vi "HW2.vi"() -> ()   [LabVIEW 2021]
panel:
  out "Key Pressed":i16
  out "turn":dbl
  out "Vref":dbl
  in  "Send value 7":dbl
  in  "Vref":dbl
  in  "Send value 8":dbl
  in  "Send value 6":dbl
  in  "Send value 5":dbl
  in  "Send value 4":dbl
  in  "Send value 3":dbl
  in  "turn":dbl
  in  "Send button":bool
  out "RecvValue 8":dbl
  out "RecvValue 7":dbl
  out "RecvValue 6":dbl
  out "RecvValue 5":dbl
  out "RecvValue 4":dbl
  out "RecvValue 3":dbl
  out "Y":dbl
  out "X":dbl
  in  "Display History":bool
  in  "Size of Rectangle":i16=20
  in  "Stop":bool
  out "2D Picture":picture
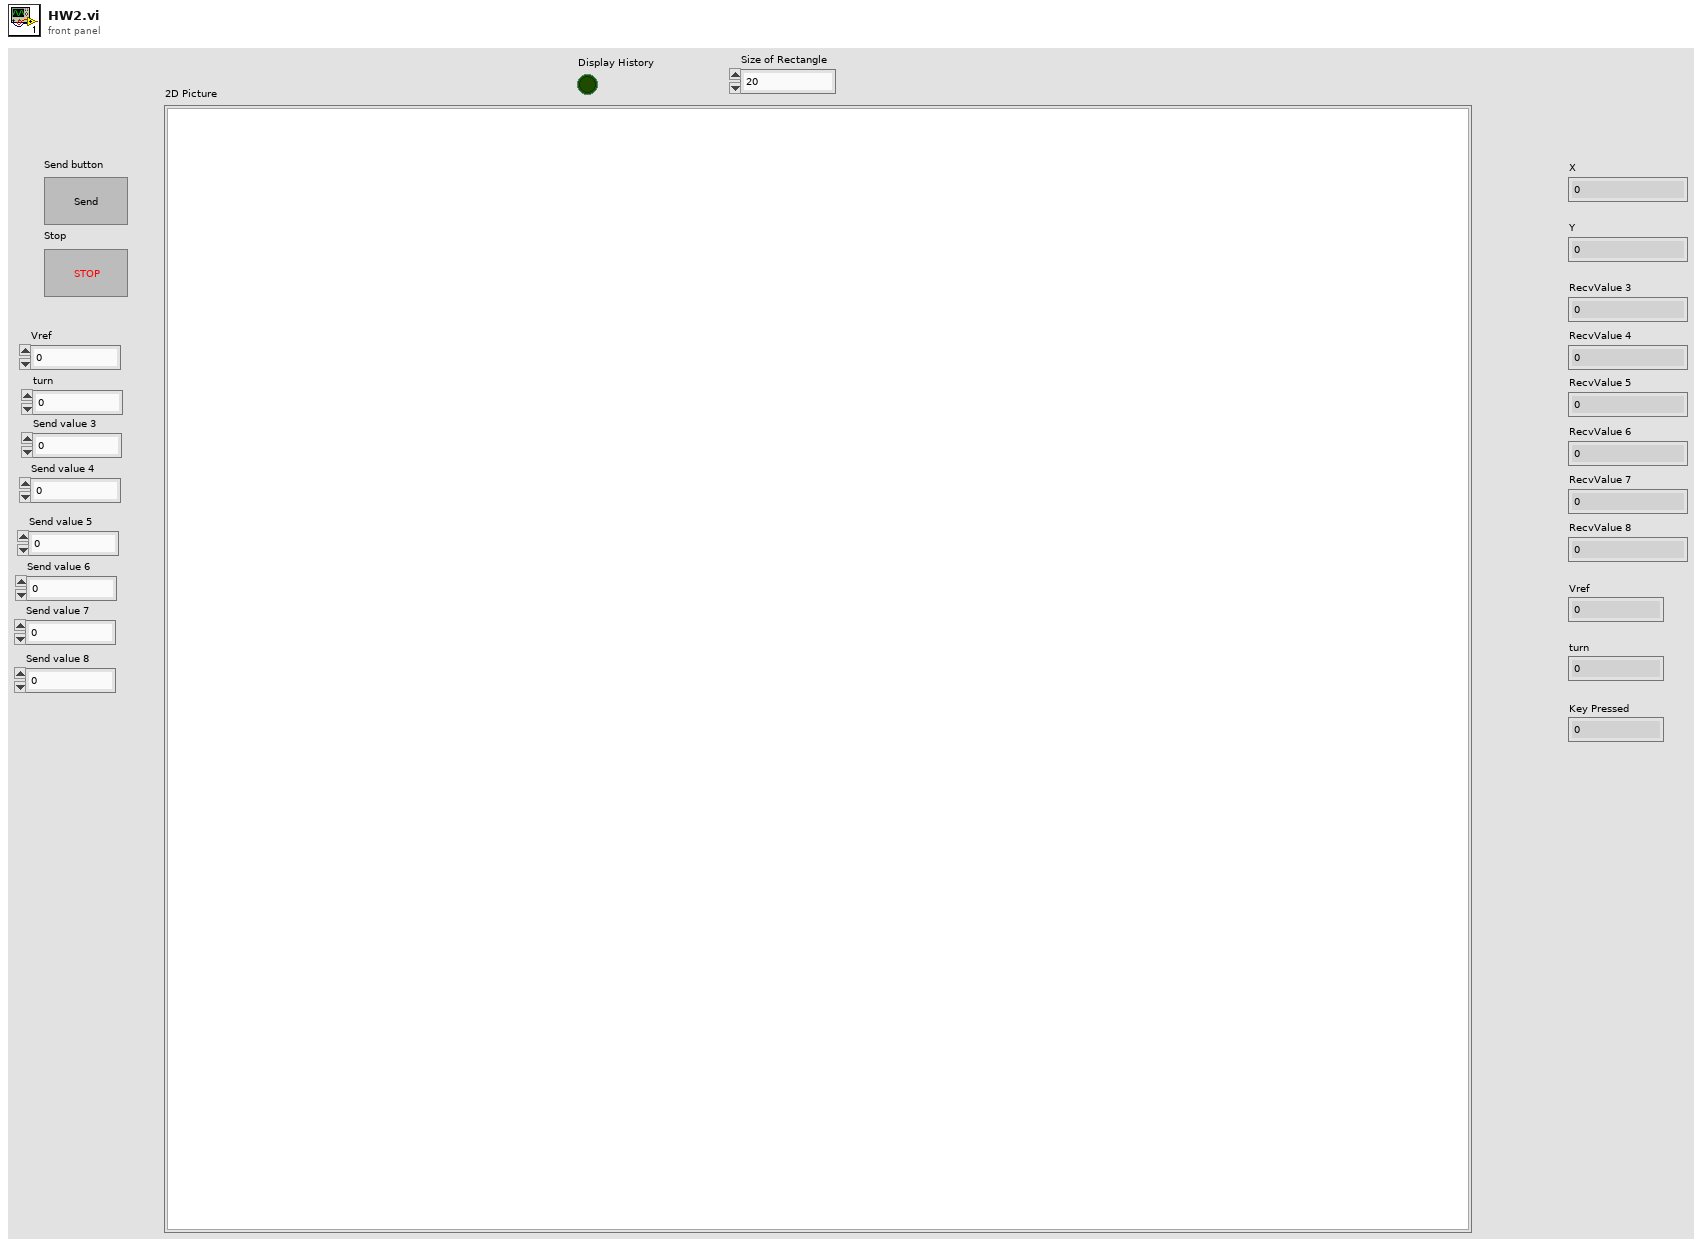
[diagram p1: front panel]
types:
  T1 = enum16{"Standard", "Buffered", "CRLF", "Immediate"}
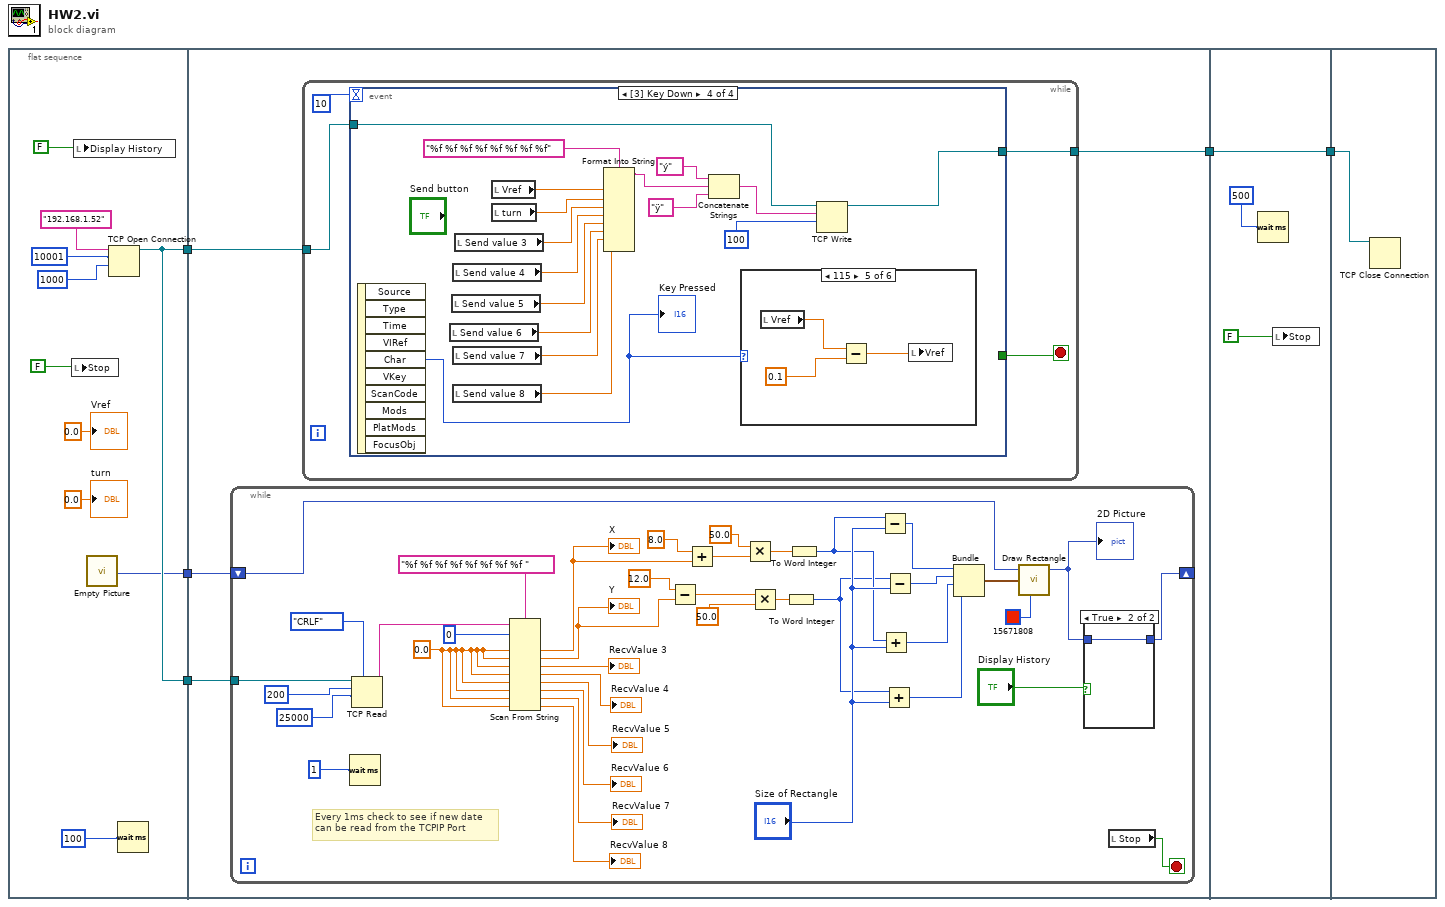
[diagram p0: block diagram]
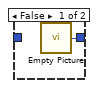
[diagram p2: hidden frame]
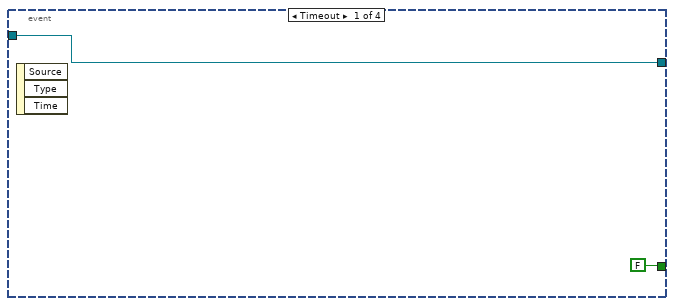
[diagram p3: hidden frame]
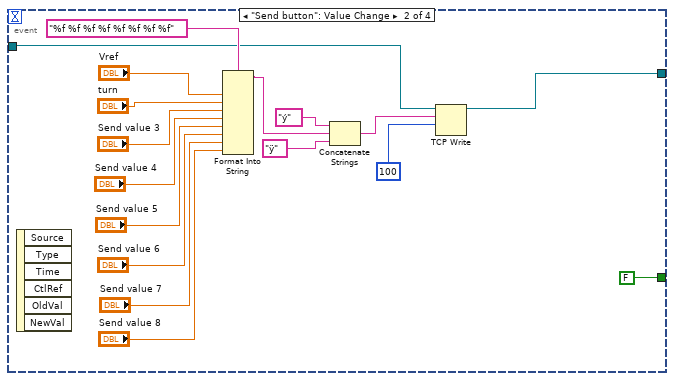
[diagram p4: hidden frame]
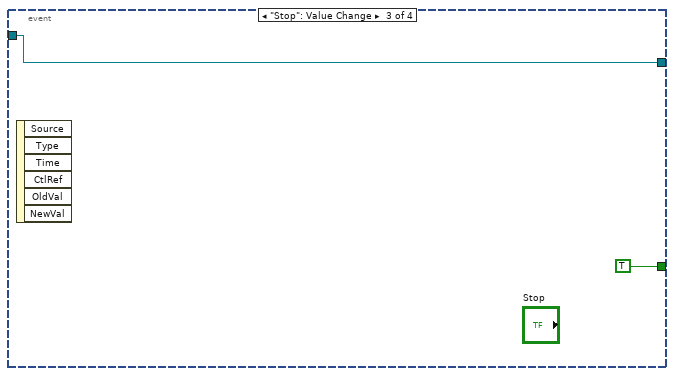
[diagram p5: hidden frame]
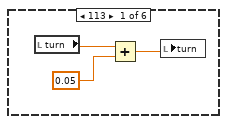
[diagram p6: hidden frame]
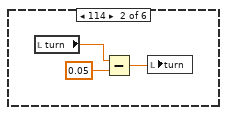
[diagram p7: hidden frame]
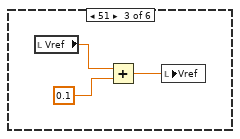
[diagram p8: hidden frame]
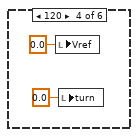
[diagram p9: hidden frame]
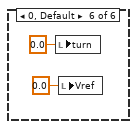
[diagram p10: hidden frame]
diagram:
  n1 = flat-sequence {
    tunnel: [w11] -> w5
    tunnel: [w11] -> w2
    tunnel: [w10] -> w1
    tunnel: w5 -> [w19]
    tunnel: [w18] -> w3
    tunnel: w2 -> [w17]
    tunnel: w1 -> [w16]
    tunnel: [w121] -> w4
    tunnel: w3 -> [w121]
    tunnel: w4 -> [w122]
    frame #0 {
      n2 = local write "Stop"(FALSE) -> ()
      n3 = local write "Display History"(FALSE) -> ()
      n4 = call "Empty Picture"() -> ("empty picture"=w10:picture)
      n5 = TCP Open Connection(address="192.168.1.52", remote port or service name=u16 10001, timeout ms (60000)=1000) -> (connection ID=w11:refnum<k5>)  [unwired: 2 in, 1 out]
      n6 = Wait (ms)(milliseconds to wait=u32 100) -> ()  [unwired: 1 out]
      "Vref" <- 0.0 ("Vref")
      "turn" <- 0.0 ("turn")
    }
    frame #1 {
      n7 = while {
        tunnel: w17 -> [w57]
        shift-right: [w24] -> _
        shift-left: w16 -> [w23]
        stop <- w21 stop-if-true
        w52 = 0.0 ("default value 1")
        # "Every 1ms check to see if new date\ncan be read from the TCPIP Port"
        n8 = Wait (ms)(milliseconds to wait=u32 1) -> ()  [unwired: 1 out]
        n9 = TCP Read(connection ID=w57, bytes to read=200, 7:T1."CRLF" ("mode (standard)"), 9:25000 ("timeout ms (25000)")) -> (data out=w53:string)  [unwired: 1 in, 2 out]
        n10 = Scan From String "Scan From String"(format string="%f %f %f %f %f %f %f %f ", input string=w53, initial scan location=u32 0, default 1=w52, default 2=w52, default 3=w52, default 4=w52, default 5=w52, default 6=w52, default 7=w52, default 8=w52) -> (output 1=w43:dbl, output 2=w41:dbl, output 3=→"RecvValue 3":dbl, output 4=→"RecvValue 4":dbl, output 5=→"RecvValue 5":dbl, output 6=→"RecvValue 6":dbl, output 7=→"RecvValue 7":dbl, output 8=→"RecvValue 8":dbl)  [unwired: 1 in, 3 out]
        "X" <- w43
        "Y" <- w41
        n11 = Subtract(x=12.0, y=w41) -> (x-y=w37:dbl)
        n12 = Add(x=8.0, y=w43) -> (x+y=w36:dbl)
        n13 = Multiply(x=50.0, y=w36) -> (x*y=w40:dbl)
        n14 = Multiply(x=w37, y=50.0) -> (x*y=w39:dbl)
        n15 = To Word Integer(number=w39) -> (16bit integer=w32:i16)
        n16 = To Word Integer(number=w40) -> (16bit integer=w33:i16)
        n17 = Subtract(x=w33, y="Size of Rectangle") -> (x-y=w31:i16)
        n18 = Add(x=w33, y="Size of Rectangle") -> (x+y=w29:i16)
        n19 = Add(x=w32, y="Size of Rectangle") -> (x+y=w28:i16)
        n20 = Subtract(x=w32, y="Size of Rectangle") -> (x-y=w30:i16)
        n21 = Bundle(w31, w30, w29, w28) -> (w27:cluster{i16, i16, i16, i16})  [unwired: 1 in]
        n22 = call <vilib>:"Draw Rectangle.vi"("picture"=w23, "rect"=w27, "color(black)"=u32 15671808) -> ("new picture"=w25:picture)  [unwired: 6 in]
        "2D Picture" <- w25
        n23 = case shown="True" "Display History" {
          tunnel: [w59 w60] -> w24
          tunnel: w25 -> [_ w60]
          frame False {
            n24 = call "Empty Picture"() -> ("empty picture"=w59:picture)
          }
          frame True {
          }
        }
        n25 = local read "Stop"() -> (w21:bool)
      }
      n26 = while {
        tunnel: w19 -> [w63]
        tunnel: [w62] -> w18
        stop <- w61 stop-if-true
        n27 = event shown="[3] Key Down" {
          selector: _ -> [_ _ _ _]
          dyn-events: _ -> [_ _ _ _]
          timeout: 10 -> [_ _ _ _]
          tunnel: w63 -> [w66 w69 w85 w96]
          tunnel: [w66 w68 w85 w97] -> w62
          tunnel: [FALSE FALSE TRUE _] -> w61
          event Timeout {
            n28 = event-data() -> ()  [unwired: 1 in, 3 out]
          }
          event "Send button": Value Change {
            n29 = event-data() -> ()  [unwired: 1 in, 6 out]
            n30 = Format Into String "Format Into String"(format string="%f %f %f %f %f %f %f %f", "Vref", "turn", "Send value 3", "Send value 4", "Send value 5", "Send value 6", "Send value 7", "Send value 8") -> (resulting string=w75:string)  [unwired: 2 in, 1 out]
            n31 = Concatenate Strings("ý" ("string"), w75, "ÿ" ("string")) -> (w70:string)
            n32 = TCP Write(connection ID=w69, data in=w70, 9:100 ("timeout ms (25000)")) -> (connection ID out=w68:refnum<k5>)  [unwired: 1 in, 2 out]
          }
          event "Stop": Value Change {
            n33 = event-data() -> ()  [unwired: 1 in, 6 out]
          }
          event Key Down {
            n34 = event-data() -> ("Char"=w86:i16)  [unwired: 1 in, 9 out]
            "Key Pressed" <- w86
            n35 = local read "Send value 6"() -> (w89:dbl)
            n36 = local read "Send value 5"() -> (w90:dbl)
            n37 = local read "Send value 4"() -> (w91:dbl)
            n38 = local read "Send value 7"() -> (w88:dbl)
            n39 = local read "Send value 8"() -> (w87:dbl)
            n40 = local read "Send value 3"() -> (w92:dbl)
            n41 = local read "Vref"() -> (w94:dbl)
            n42 = local read "turn"() -> (w93:dbl)
            n43 = Format Into String "Format Into String"(format string="%f %f %f %f %f %f %f %f", w94, w93, w92, w91, w90, w89, w88, w87) -> (resulting string=w102:string)  [unwired: 2 in, 1 out]
            n44 = Concatenate Strings("ý" ("string"), w102, "ÿ" ("string")) -> (w98:string)
            n45 = case shown="115" w86 {
              frame 113 {
                n46 = local read "turn"() -> (w105:dbl)
                n47 = Add(x=w105, y=0.05) -> (x+y=w103:dbl)
                n48 = local write "turn"(w103) -> ()
              }
              frame 114 {
                n49 = local read "turn"() -> (w106:dbl)
                n50 = Subtract(x=w106, y=0.05) -> (x-y=w108:dbl)
                n51 = local write "turn"(w108) -> ()
              }
              frame 51 {
                n52 = local read "Vref"() -> (w110:dbl)
                n53 = Add(x=w110, y=0.1) -> (x+y=w111:dbl)
                n54 = local write "Vref"(w111) -> ()
              }
              frame 120 {
                n55 = local write "Vref"(0.0 ("Vref")) -> ()
                n56 = local write "turn"(0.0 ("turn")) -> ()
              }
              frame 115 {
                n57 = local read "Vref"() -> (w116:dbl)
                n58 = Subtract(x=w116, y=0.1) -> (x-y=w114:dbl)
                n59 = local write "Vref"(w114) -> ()
              }
              frame 0, Default {
                n60 = local write "turn"(0.0 ("turn")) -> ()
                n61 = local write "Vref"(0.0 ("Vref")) -> ()
              }
            }
            n62 = TCP Write(connection ID=w96, data in=w98, 9:100 ("timeout ms (25000)")) -> (connection ID out=w97:refnum<k5>)  [unwired: 1 in, 2 out]
          }
        }
      }
    }
    frame #2 {
      n63 = Wait (ms)(milliseconds to wait=u32 500) -> ()  [unwired: 1 out]
      n64 = local write "Stop"(FALSE) -> ()
    }
    frame #3 {
      n65 = TCP Close Connection(connection ID=w122) -> ()  [unwired: 2 in, 2 out]
    }
  }
